vi "Format Data by Type for Data Entry Field Display.vi"(1 "Test Parameters Table":i32, 2 "Cluster":T1, 3 "MCListbox Refnum":refnum<vi>) -> (0 "array type (2D Dbl)":dbl[][](array[numeric]))   [LabVIEW 2012, in "Core SubVIs.lvlib"]
uses:
  Core SubVIs.lvlib
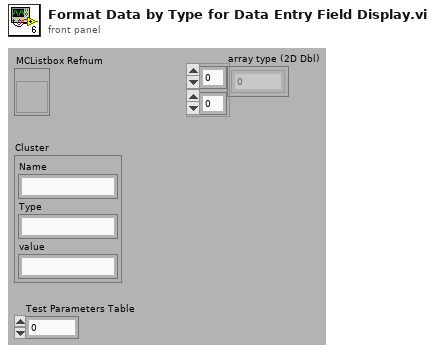
[diagram p1: front panel]
types:
  T1 = cluster{"Name":string, "Type":string, "value":string}
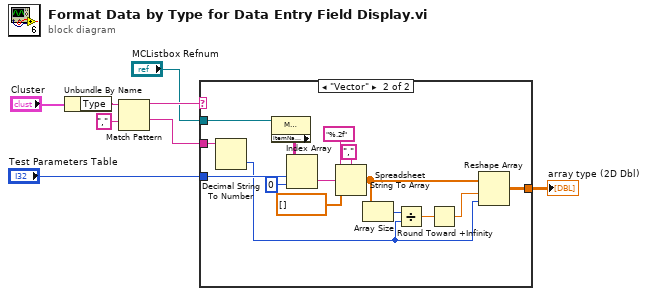
[diagram p0: block diagram]
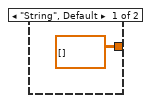
[diagram p2: hidden frame]
diagram:
  n1 = Unbundle By Name("Cluster") -> ("Type"=w4:string)
  n2 = Match Pattern(string=w4, regular expression=",") -> (before substring=w6:string, after substring=w7:string)  [unwired: 3 out]
  n3 = case shown="\"Vector\"" w6 {
    tunnel: "Test Parameters Table" -> [_ w18]
    tunnel: w7 -> [_ w15]
    tunnel: [dbl[][] [] ("array type (2D Dbl)") w17] -> w8
    tunnel: "MCListbox Refnum" -> [_ w16]
    frame "String", Default {
    }
    frame "Vector" {
      n4 = Decimal String To Number(string=w15) -> (number=w12:i32)  [unwired: 3 out]
      n5 = property on="Property Node" class="MCListbox (strict)"(reference=w16) -> ("ItemNames"=w24:string[][])  [unwired: 1 in, 2 out]
      n6 = Index Array(array=w24, index (row)=w18, index (col)=0 ("disabled index (col)")) -> (element=w22:string)
      n7 = Spreadsheet String To Array(delimiter (Tab)=",", format string="%.2f", spreadsheet string=w22, array type (2D Dbl)=dbl[] []) -> (array=w14:dbl[])
      n8 = Array Size(array=w14) -> (size(s)=w13:i32)
      n9 = Divide(x=w13, y=w12) -> (x/y=w11:dbl)
      n10 = Round Toward +Infinity(x=w11) -> (ceil(x): smallest int >= x=w10:dbl)
      n11 = Reshape Array(w14, w10, w12) -> (w17:dbl[][])
    }
  }
  "array type (2D Dbl)" <- w8
